vi "Cumulative Time Calculator for Testing Log.vi"(8 "error in (no error)":errorcluster, 11 "Input Matrix":T1) -> (0 "error out":errorcluster, 3 "Output Matrix":T1)   [LabVIEW 2010]
uses:
  <vilib>/Analysis/Matrix/Datatypes/RealMatrix.ctl
  <vilib>/Analysis/Matrix/NI_Matrix.lvlib
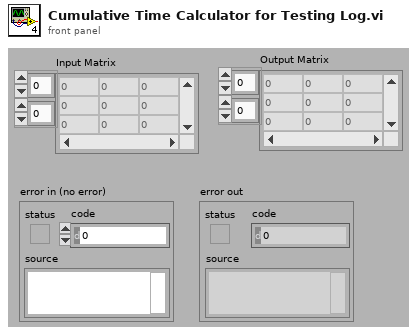
[diagram p1: front panel]
types:
  T1 = typedef "NI_Matrix.lvlib/RealMatrix.ctl" = dbl[][]
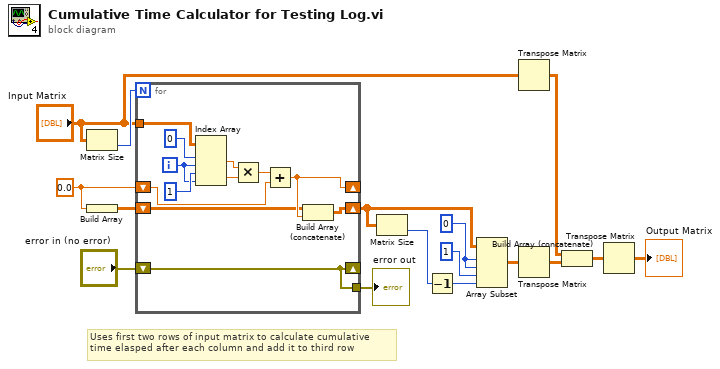
[diagram p0: block diagram]
diagram:
  w13 = 0
  w15 = 0.0
  # "Uses first two rows of input matrix to calculate cumulative\ntime elasped after each column and add it to third row"
  n1 = Matrix Size(0:"Input Matrix") -> (2:w16:i32)  [unwired: 1 out]
  n2 = Build Array(w15) -> (w14:T1)
  n3 = for {
    N: w16 -> [_]
    tunnel: "Input Matrix" -> [w26]
    shift-right: [w18] -> _
    shift-left: w15 -> [w21]
    shift-right: [w20] -> w9
    shift-left: w14 -> [w17]
    shift-right: [w19] -> _
    shift-left: "error in (no error)" -> [w19]
    tunnel: [w19] -> w7
    i -> [w25]
    n4 = Index Array(array=w26, index (row) #1=0, index (col) #1=w25, index (row) #2=1, index (col) #2=w25) -> (element #1=w24:dbl, element #2=w23:dbl)
    n5 = Multiply(x=w24, y=w23) -> (x*y=w22:dbl)
    n6 = Add(x=w22, y=w21) -> (x+y=w18:dbl)
    n7 = Build Array (concatenate)(w17, w18) -> (w20:T1)
  }
  "error out" <- w7
  n8 = Matrix Size(0:w9) -> (2:w11:i32)  [unwired: 1 out]
  n9 = Decrement(x=w11) -> (x-1=w10:i32)
  n10 = Array Subset(array=w9, index (row)=w13, length (row)=w13, index (col)=1, length (col)=w10) -> (w2:T1)
  n11 = Transpose Matrix(1:"Input Matrix") -> (0:w5:T1)
  n12 = Transpose Matrix(1:w2) -> (0:w1:T1)
  n13 = Build Array (concatenate)(w5, w1) -> (w4:T1)
  n14 = Transpose Matrix(1:w4) -> (0:→"Output Matrix":T1)
